vi "Update System Status.vi"(0 "system status ctl ref in":refnum<vi>, 5 "system status in":string, 11 "error in":errorcluster) -> (15 "error out":errorcluster)   [LabVIEW 2016, in "TLB` Template.lvlib"]
doc: "Update current system status.\n\n<B>Input Parameters</B>\n\n<B>system status in</B> system status control reference.\n\n<B>system status message</B> is the current system status.\n\n<B>error in</B> describes error conditions that occur before this node runs. This input provides standard error in functionality. \n\n<B>Output Parameters</B>\n\n<B>error out</B> contains error information. This output provides standard error out functionality."
uses:
  TLB` Template.lvlib
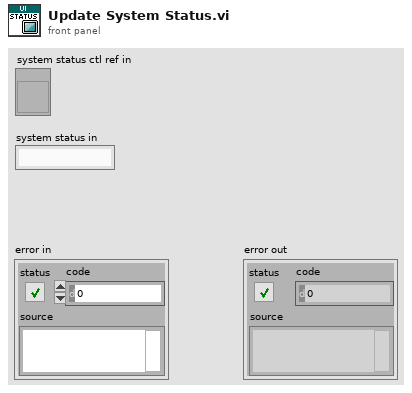
[diagram p1: front panel]
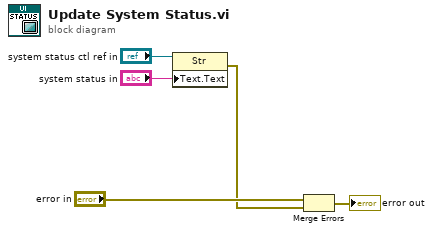
[diagram p0: block diagram]
diagram:
  n1 = property class="Str"(reference="system status ctl ref in", "Text.Text"="system status in") -> (error out=w3:errorcluster)  [unwired: 1 in, 1 out]
  n2 = Merge Errors("error in", w3) -> (→"error out":errorcluster)
